vi "Shot Overlay (SubVI).vi"(7 "Image Out":T1, 8 "Particle Measurements (Pixels) (Particle Analysis 1)":dbl[][](array[numeric]), 9 "Particle Measurements (Real-World) (Particle Analysis 1)":dbl[][](array[numeric]), 10 "Nb Circles (Circle Detection 1)":i32) -> (1 "Image Out 2":T1, 2 "Player Position Pixels":dbl[][](array[numeric]), 3 "Puck position pixels":dbl[][](array[numeric]))   [LabVIEW 2013]
uses:
  <vilib>/vision/Image Controls.llb/IMAQ Image.ctl
panel:
  out "output cluster":cluster{i32, i32, i32, i32}
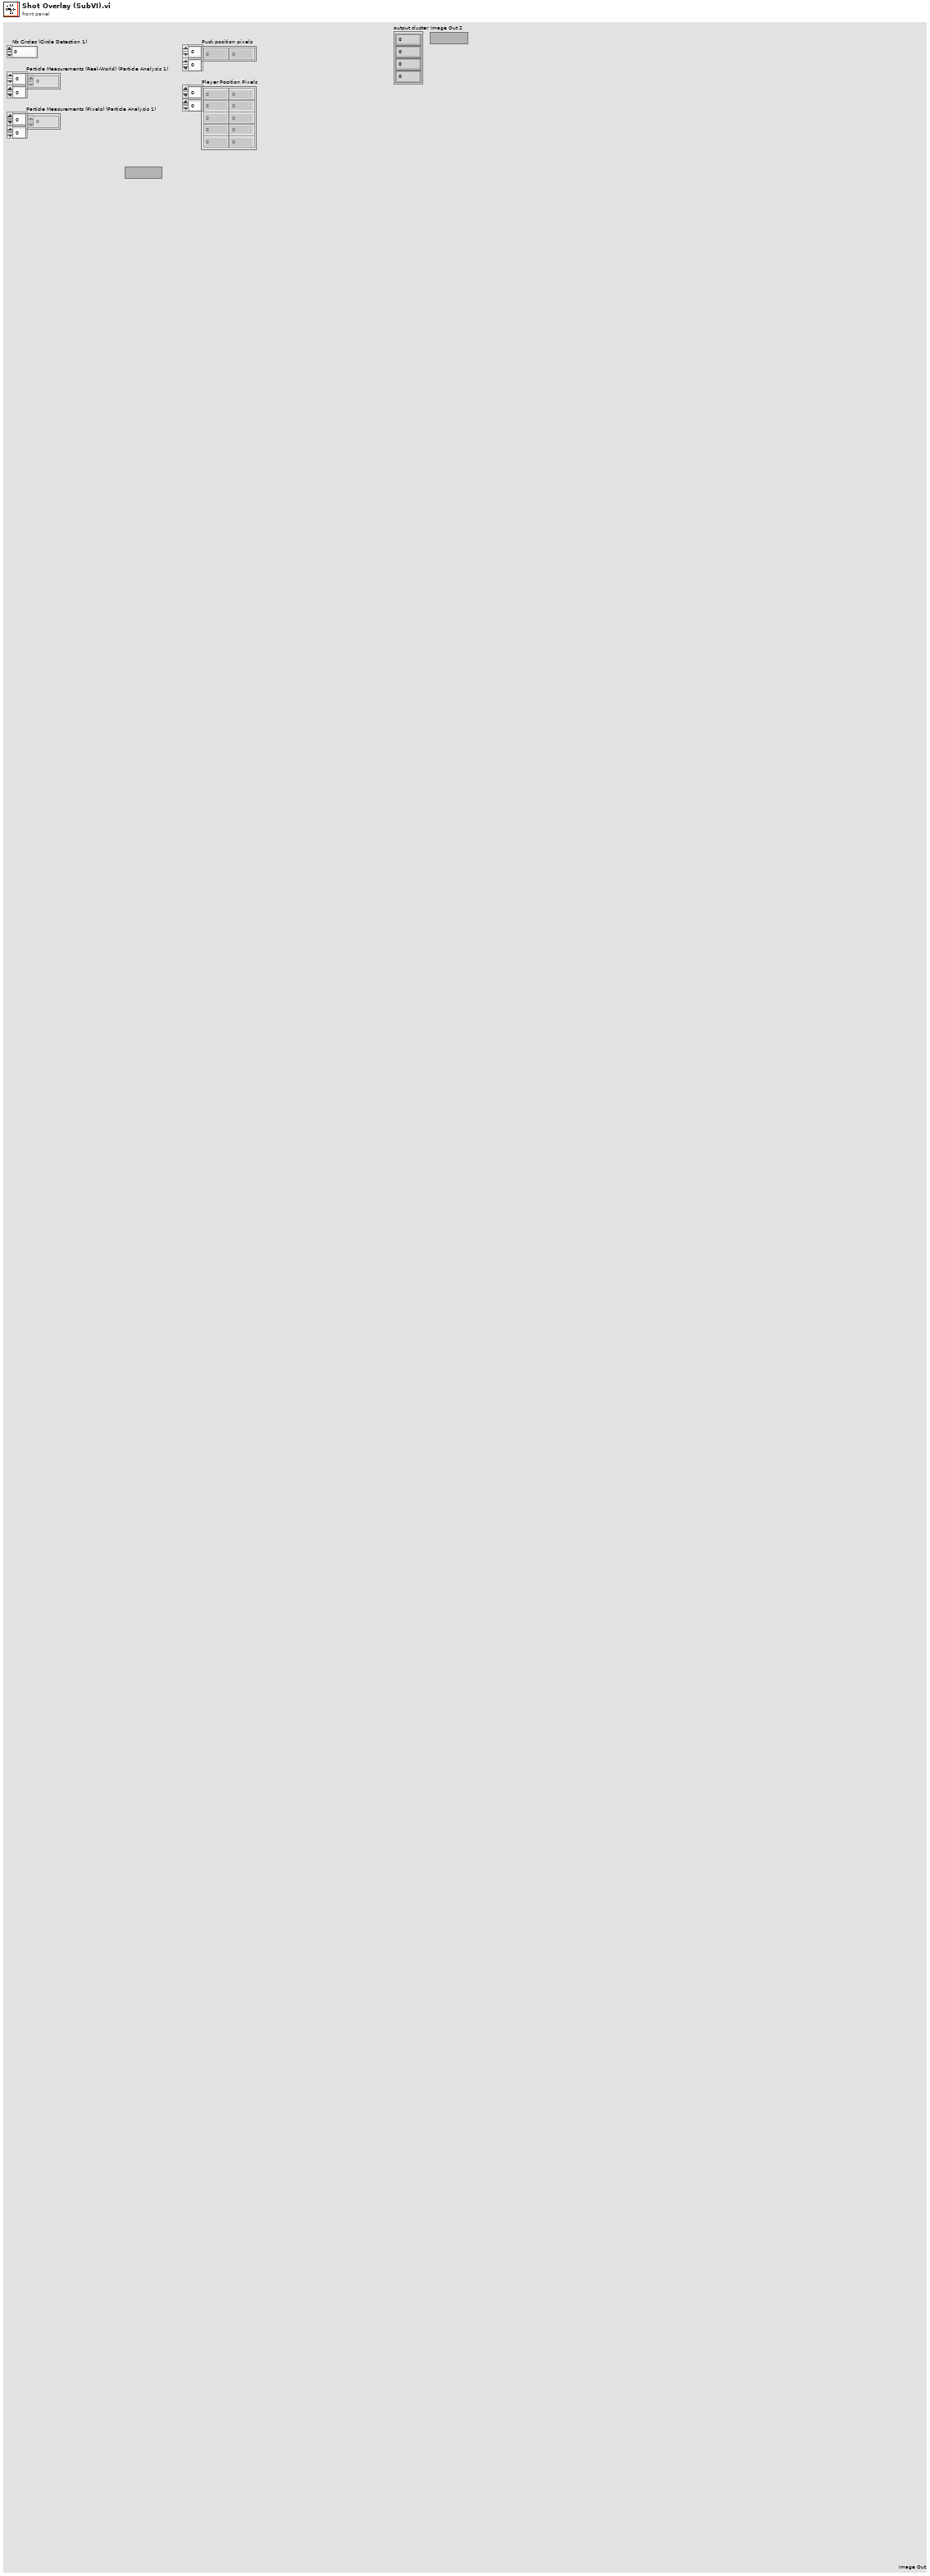
[diagram p1: front panel]
types:
  T1 = typedef "IMAQ Image.ctl" = refnum<image>
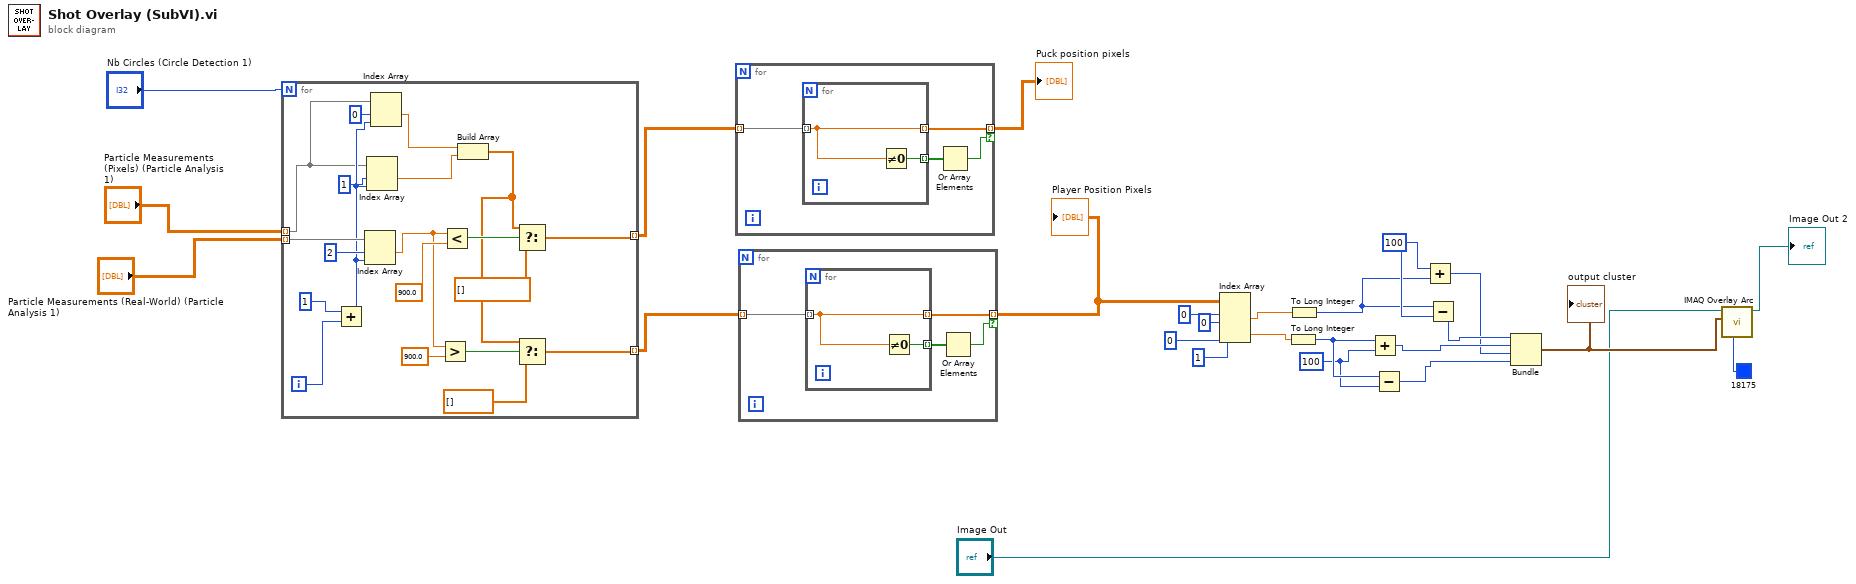
[diagram p0: block diagram]
diagram:
  w9 = 100 ("y")
  w14 = 100 ("x")
  n1 = for {
    N: "Nb Circles (Circle Detection 1)" -> [_]
    tunnel: "Particle Measurements (Real-World) (Particle Analysis 1)" -> [w38] mode=indexing
    tunnel: [w40] -> w21 mode=indexing
    tunnel: [w27] -> w22 mode=indexing
    tunnel: "Particle Measurements (Pixels) (Particle Analysis 1)" -> [w26] mode=indexing
    i -> [w44]
    n2 = Add(x=1, y=w44) -> (x+y=w36:i32)
    n3 = Index Array(array=w38, index #1=2 ("index"), index #2=w36) -> (element #1=w31:dbl)  [unwired: 1 out]
    n4 = Index Array(array=w26, index #1=1 ("index"), index #2=w36) -> (element #1=w34:dbl)  [unwired: 1 out]
    n5 = Index Array(array=w26, index #1=0 ("index"), index #2=w36) -> (element #1=w35:dbl)  [unwired: 1 out]
    n6 = Greater?(x=w31, y=900.0) -> (0:w30:bool)
    n7 = Less?(x=w31, y=900.0) -> (x < y?=w41:bool)
    n8 = Build Array(w35, w34) -> (w29:dbl[])
    n9 = Select(t=w29, s=w41, f=dbl[] []) -> (s? t:f=w40:dbl[])
    n10 = Select(t=w29, s=w30, f=dbl[] []) -> (s? t:f=w27:dbl[])
  }
  n11 = for {
    tunnel: w21 -> [w49] mode=indexing
    tunnel: [w47] -> w25 mode=indexing if=w46
    n12 = for {
      tunnel: w49 -> [w50] mode=indexing
      tunnel: [w51] -> w48 mode=indexing
      tunnel: [w50] -> w47 mode=indexing
      n13 = Not Equal To 0?(x=w50) -> (x != 0?=w51:bool)
    }
    n14 = Or Array Elements(Boolean array=w48) -> (logical OR=w46:bool)
  }
  "Puck position pixels" <- w25
  n15 = for {
    tunnel: w22 -> [w55] mode=indexing
    tunnel: [w53] -> w19 mode=indexing if=w52
    n16 = for {
      tunnel: w55 -> [w56] mode=indexing
      tunnel: [w57] -> w54 mode=indexing
      tunnel: [w56] -> w53 mode=indexing
      n17 = Not Equal To 0?(x=w56) -> (x != 0?=w57:bool)
    }
    n18 = Or Array Elements(Boolean array=w54) -> (logical OR=w52:bool)
  }
  "Player Position Pixels" <- w19
  n19 = Index Array(array=w19, index (row) #1=0 ("index (row)"), index (col) #1=0 ("disabled index (col)"), index (row) #2=0 ("index (row)"), index (col) #2=1 ("disabled index (col)")) -> (element #1=w13:dbl, element #2=w11:dbl)
  n20 = To Long Integer(number=w11) -> (32bit integer=w10:i32)
  n21 = To Long Integer(number=w13) -> (32bit integer=w12:i32)
  n22 = Add(x=w10, y=w9) -> (x+y=w7:i32)
  n23 = Subtract(x=w10, y=w9) -> (x-y=w5:i32)
  n24 = Add(x=w14, y=w12) -> (x+y=w6:i32)
  n25 = Subtract(x=w12, y=w14) -> (x-y=w8:i32)
  n26 = Bundle(w8, w7, w6, w5) -> (w3:cluster{i32, i32, i32, i32})  [unwired: 1 in]
  "output cluster" <- w3
  n27 = call "IMAQ Overlay Arc"("Color"=u32 18175, "Bounding Rectangle"=w3, "Image"="Image Out") -> ("Image Out"=→"Image Out 2":T1)  [unwired: 7 in, 1 out]
